vi "Determine Window Position.vi"(9 "Window Bounds":T1, 10 "On Right?":bool, 11 "Position":cluster{"Left":i32, "Top":i32}) -> (3 "Window Bounds":T1)   [LabVIEW 2020, in "Peek Window.lvlib"]
uses:
  Peek Window.lvlib
  <vilib>/Utility/miscctls.llb/LVRectTypeDef.ctl
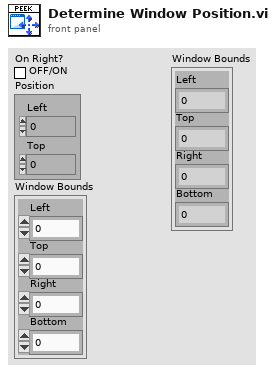
[diagram p1: front panel]
types:
  T1 = typedef "LVRectTypeDef.ctl" = cluster{"Left":i16, "Top":i16, "Right":i16, "Bottom":i16}
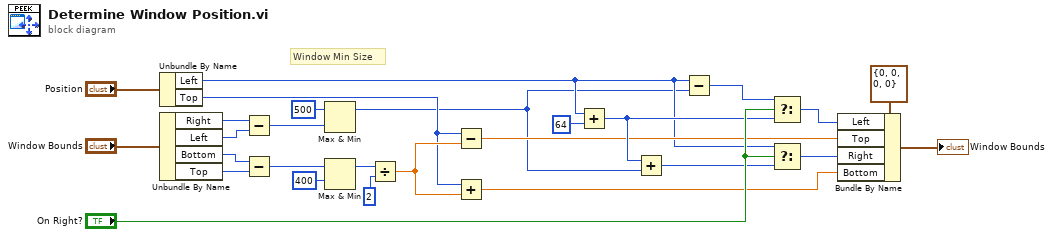
[diagram p0: block diagram]
diagram:
  # "Window Min Size"
  n1 = Unbundle By Name("Position") -> ("Left"=w9:i32, "Top"=w8:i32)
  n2 = Unbundle By Name("Window Bounds") -> ("Right"=w6:i16, "Left"=w12:i16, "Bottom"=w13:i16, "Top"=w7:i16)
  n3 = Subtract(x=w6, y=w12) -> (x-y=w24:i16)
  n4 = Subtract(x=w13, y=w7) -> (x-y=w2:i16)
  n5 = Max & Min(x=i16 500, y=w24) -> (max(x,y)=w4:i16)  [unwired: 1 out]
  n6 = Max & Min(x=w2, y=i16 400 ("x")) -> (max(x,y)=w3:i16)  [unwired: 1 out]
  n7 = Divide(x=w3, y=i16 2) -> (x/y=w17:dbl)
  n8 = Subtract(x=w8, y=w17) -> (x-y=w18:dbl)
  n9 = Add(x=w8, y=w17) -> (x+y=w19:dbl)
  n10 = Add(x=w9, y=64 ("x")) -> (x+y=w23:i32)
  n11 = Add(x=w23, y=w4) -> (x+y=w22:i32)
  n12 = Subtract(x=w9, y=w4) -> (x-y=w25:i32)
  n13 = Select(t=w25, s="On Right?", f=w23) -> (s? t:f=w26:i32)
  n14 = Select(t=w9, s="On Right?", f=w22) -> (s? t:f=w21:i32)
  n15 = Bundle By Name(cluster=T1 {"Left"=0, "Top"=0, "Right"=0, "Bottom"=0} ("Front Panel Window:Window Bounds"), "Left"=w26, "Top"=w18, "Right"=w21, "Bottom"=w19) -> (→"Window Bounds":T1)
